vi "test.vi"() -> ()   [LabVIEW 2012]
panel:
  out "Numeric 2":dbl
  out "Numeric":dbl
  in  "test1":dbl[unit]
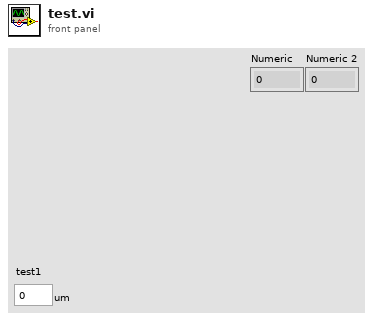
[diagram p1: front panel]
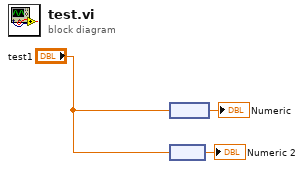
[diagram p0: block diagram]
diagram:
  n1 = node("test1") -> (→"Numeric":dbl)
  n2 = node("test1") -> (→"Numeric 2":dbl)
